vi "Define axes to command from boolean array.vi"(1 "Command axis? (num)":dbl[](array[numeric]), 2 "Axes to query":string[](array[string]), 3 "Command axis?":bool[](array[boolean]), 4 "Command axis? format\n(Boolean: FALSE)":bool) -> (14 "Axes to command":string[](array[string]), 15 "Remaining axes":string[](array[string]), 16 "Command axis? out":bool[](array[boolean]))   [LabVIEW 2026]
doc: "This VI returns only those axes IDs from the Axes to query array in the Axes to command array which have a boolean value TRUE in the Command axis? array or a numerical value of 1 in the Command axis? (num) array, depending on Command axis? format, and returns all remaining axes in the Remaining axes array."
panel:
  # "This vi returns only those axes IDs from the \"Axes to query\" array in the \"Axes to command\" array which have a \nboolean value TRUE in the \"Command axis?\" array or a numerical value of 1 in the \"Command axis? (num)\" array, \ndepending on \"Command axis? format\", and returns all remaining axes in the \"Remaining axes\" array."
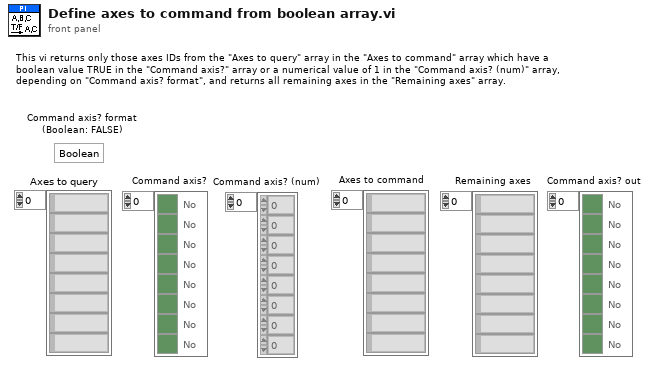
[diagram p1: front panel]
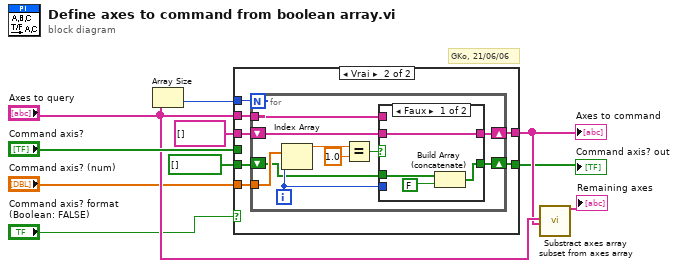
[diagram p0: block diagram]
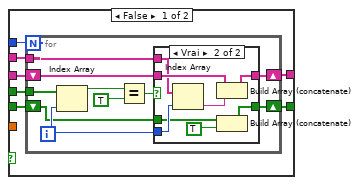
[diagram p2: hidden frame]
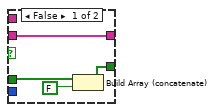
[diagram p3: hidden frame]
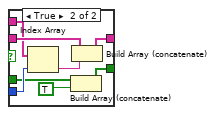
[diagram p4: hidden frame]
diagram:
  # "GKo, 21/06/06"
  n1 = Array Size(array="Axes to query") -> (size(s)=w10:i32)
  n2 = case shown="Vrai" "Command axis? format\n(Boolean: FALSE)" {
    tunnel: w10 -> [w17 w46]
    tunnel: string[] [] -> [w16 w45]
    tunnel: "Command axis?" -> [w15 _]
    tunnel: "Axes to query" -> [w14 w44]
    tunnel: [w13 w43] -> w6
    tunnel: "Command axis? (num)" -> [_ w42]
    tunnel: bool[] [] ("Command axis?") -> [w12 w41]
    tunnel: [w11 w40] -> w1
    frame False {
      n3 = for {
        N: w17 -> [_]
        tunnel: w15 -> [w26]
        shift-right: [w24] -> w13
        shift-left: w16 -> [w23]
        tunnel: w14 -> [w22]
        shift-right: [w19] -> w11
        shift-left: w12 -> [w18]
        i -> [w21]
        n4 = Index Array(array=w26, index=w21) -> (element=w27:bool)
        n5 = Equal?(x=w27, y=TRUE) -> (x = y?=w20:bool)
        n6 = case shown="Vrai" w20 {
          tunnel: [w31 w39] -> w24
          tunnel: w23 -> [w31 w38]
          tunnel: w22 -> [_ w36]
          tunnel: w21 -> [_ w35]
          tunnel: [w28 w34] -> w19
          tunnel: w18 -> [w29 w33]
          frame False {
            n7 = Build Array (concatenate)(w29, FALSE) -> (w28:bool[])
          }
          frame True {
            n8 = Index Array(array=w36, index=w35) -> (element=w37:string)
            n9 = Build Array (concatenate)(w38, w37) -> (w39:string[])
            n10 = Build Array (concatenate)(w33, TRUE) -> (w34:bool[])
          }
        }
      }
    }
    frame True {
      n11 = for {
        N: w46 -> [_]
        shift-right: [w55] -> w43
        shift-left: w45 -> [w54]
        tunnel: w44 -> [w53]
        tunnel: w42 -> [w50]
        shift-right: [w48] -> w40
        shift-left: w41 -> [w47]
        i -> [w52]
        n12 = Index Array(array=w50, index=w52) -> (element=w56:dbl)
        n13 = Equal?(x=w56, y=1.0) -> (x = y?=w51:bool)
        n14 = case shown="Faux" w51 {
          tunnel: [w60 w68] -> w55
          tunnel: w54 -> [w60 w67]
          tunnel: w53 -> [_ w65]
          tunnel: w52 -> [_ w64]
          tunnel: [w57 w63] -> w48
          tunnel: w47 -> [w59 w62]
          frame False {
            n15 = Build Array (concatenate)(w59, FALSE) -> (w57:bool[])
          }
          frame True {
            n16 = Index Array(array=w65, index=w64) -> (element=w66:string)
            n17 = Build Array (concatenate)(w62, TRUE) -> (w63:bool[])
            n18 = Build Array (concatenate)(w67, w66) -> (w68:string[])
          }
        }
      }
    }
  }
  "Axes to command" <- w6
  "Command axis? out" <- w1
  n19 = call "Substract axes array subset from axes array.vi"("Axes to query"="Axes to query", "Axes subset"=w6) -> ("Axes to command"=→"Remaining axes":string[])  [unwired: 1 in, 16 out]
